vi "Write Configuration.lvlib_Configuration.lvclass.vi"(8 "error in (no error)":errorcluster, 10 "Hardware.lvlib:HW Configuration.lvclass":refnum<class "HW Configuration.lvclass">, 11 "Hardware in":refnum<class "Hardware.lvclass">) -> (0 "error out":errorcluster, 3 "Hardware out":refnum<class "Hardware.lvclass">)   [LabVIEW 2017, in "Hardware.lvlib" / "Hardware.lvclass"]
uses:
  Hardware.lvclass
  HW Config/HW Configuration.lvclass
  Hardware.lvclass/Hardware.ctl
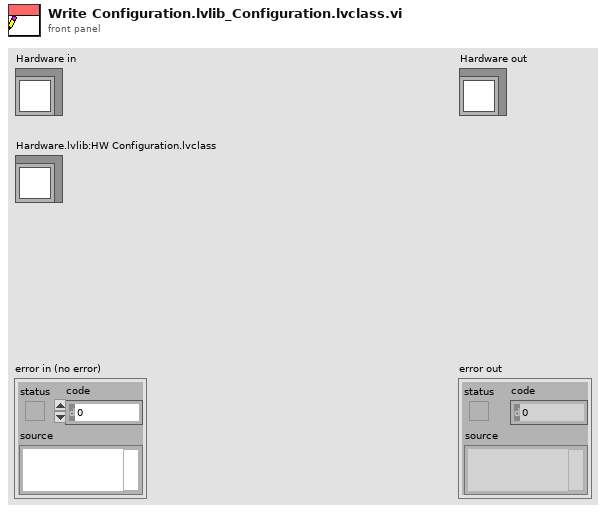
[diagram p1: front panel]
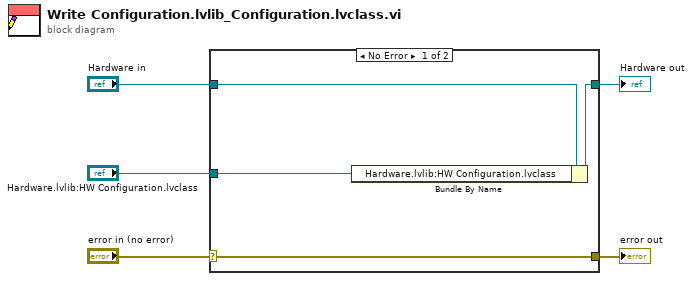
[diagram p0: block diagram]
diagram:
  n1 = case shown="No Error" "error in (no error)" {
    selector: "error in (no error)" -> [w9 w10]
    tunnel: [w9 w10] -> w4
    tunnel: [w8 w11] -> w2
    tunnel: "Hardware in" -> [w6 w11]
    tunnel: "Hardware.lvlib:HW Configuration.lvclass" -> [w7 _]
    frame No Error {
      n2 = Bundle By Name(cluster=w6, "Hardware.lvlib:HW Configuration.lvclass"=w7) -> (w8:refnum<class "Hardware.lvclass">)
    }
    frame Error {
    }
  }
  "error out" <- w4
  "Hardware out" <- w2
